vi "data insert core.vi"(8 "error in (no error)":errorcluster, 9 "column information":T1[](array[typedef]), 10 "data":variant[](array[variant]), 11 "table":string) -> (0 "error out":errorcluster)   [LabVIEW 2016, in "斯坦道多参数.lvlib"]
uses:
  <vilib>/addons/database/Auxilliary.llb/DB Tools Column Info.ctl
  <vilib>/addons/database/Auxilliary.llb/DB Tools DataTypes.ctl
  <vilib>/Utility/sysdir.llb/System Directory Type.ctl
  <vilib>/addons/database/Auxilliary.llb/DB Tools Transaction.ctl
  <vilib>/addons/database/Auxilliary.llb/DB Tools Isolation Level.ctl
  <vilib>/addons/database/Auxilliary.llb/DB Tools Parameter Info.ctl
  <vilib>/addons/database/Auxilliary.llb/DB Tools Parameter Dir.ctl
  <vilib>/addons/database/Connection.llb/DB Tools Open Connec (String).vi
  <vilib>/addons/database/Connection.llb/Conn Transaction.vi
  <vilib>/addons/database/Connection.llb/Conn Execute.vi
  <vilib>/addons/database/Recordset.llb/Rec Destroy - Connection.vi
  <vilib>/addons/database/Command.llb/Cmd Set Parameter Value (C).vi
  <vilib>/addons/database/Auxilliary.llb/DB Tools Format Datetime String (Time Stamp).vi
  <vilib>/addons/database/Command.llb/Cmd Execute.vi
  <vilib>/addons/database/Recordset.llb/Rec Destroy - Command.vi
  <vilib>/addons/database/Command.llb/Cmd Delete.vi
  <vilib>/addons/database/NI_Database_API.lvlib
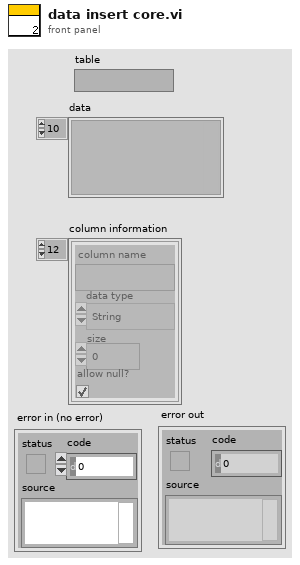
[diagram p1: front panel]
types:
  T1 = typedef "NI_Database_API.lvlib/DB Tools Column Info.ctl" = cluster{"column name":string, "data type":T2, "size":i32, "allow null?":bool}
  T2 = typedef "NI_Database_API.lvlib/DB Tools DataTypes.ctl" = enum16{"String", "Long (I32)", "Single (SGL)", "Double (DBL)", "Date/Time", "Binary"}
  T3 = typedef "NI_Database_API.lvlib/DB Tools Isolation Level.ctl" = enum16{"chaos", "read uncommitted", "read committed", "repeatable read", "serializable"}
  T4 = typedef "NI_Database_API.lvlib/DB Tools Transaction.ctl" = enum16{"begin", "commit", "rollback"}
  T5 = typedef "System Directory Type.ctl" = i32
  T6 = typedef "NI_Database_API.lvlib/Conn ObjectReference.ctl" = refnum<k1>
  T7 = typedef "NI_Database_API.lvlib/DB Tools Parameter Info.ctl" = cluster{"parameter name":string, "type":T2, "direction":T8, "value":variant}
  T8 = typedef "NI_Database_API.lvlib/DB Tools Parameter Dir.ctl" = enum32{"Input", "Output", "Input/Output", "Return Value"}
  T9 = typedef "NI_Database_API.lvlib/Rec ObjectReference.ctl" = refnum<k1>
  T10 = typedef "NI_Database_API.lvlib/Cmd ObjectReference.ctl" = refnum<k1>
  T11 = typedef "NI_Database_API.lvlib/Cmd-Rec Object Reference.ctl" = refnum<k1>
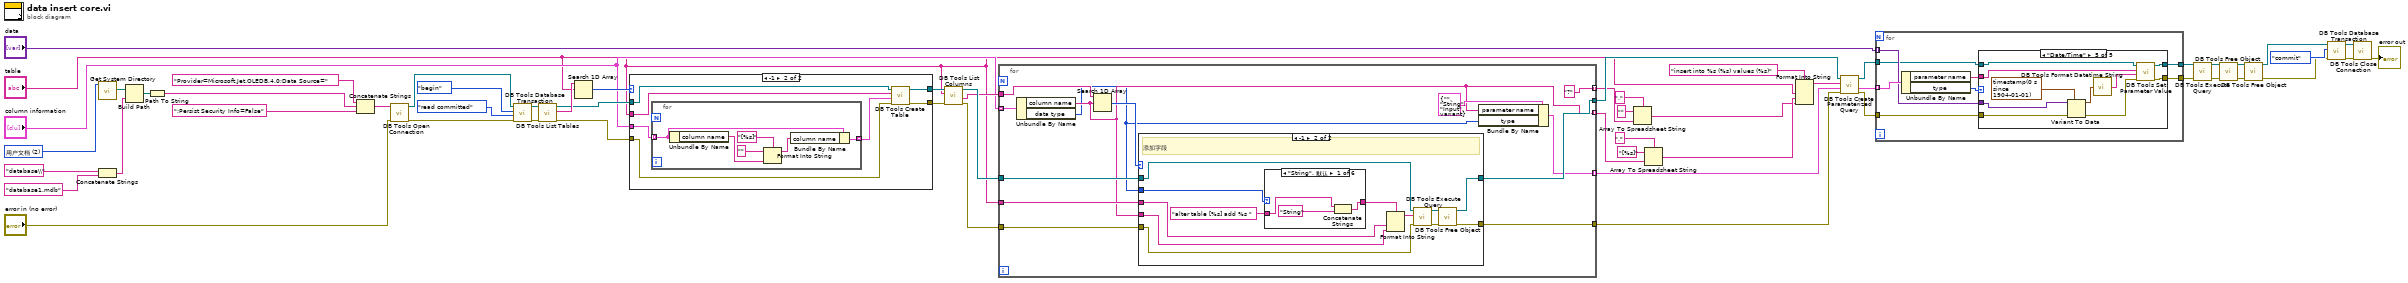
[diagram p0: block diagram]
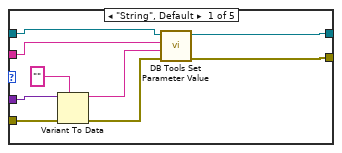
[diagram p2: hidden frame]
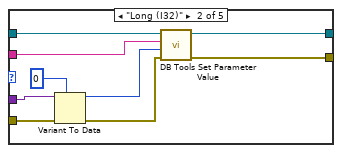
[diagram p3: hidden frame]
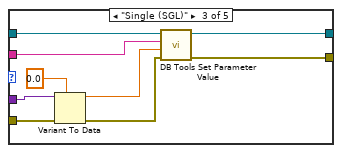
[diagram p4: hidden frame]
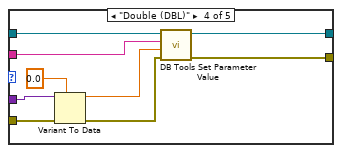
[diagram p5: hidden frame]
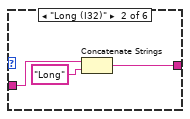
[diagram p7: hidden frame]
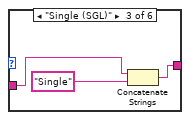
[diagram p8: hidden frame]
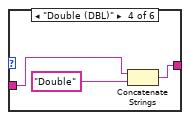
[diagram p9: hidden frame]
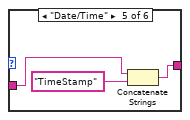
[diagram p10: hidden frame]
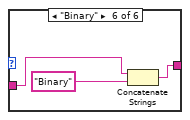
[diagram p11: hidden frame]
diagram:
  w57 = T5 2 items=["用户目录"=0, "用户桌面"=1, "用户文档"=2, "用户应用程序数据"=3, "用户设置"=4, "用户临时目录"=5, "公共文档"=6, "公共应用程序数据"=7, "公共设置"=8, "公共缓存"=13, "系统核心库"=9, "系统安装库"=10, "应用程序文件"=11, "启动盘根目录"=12] ("system directory type")
  n1 = call <vilib>:"Get System Directory.vi"("system directory type"=w57) -> ("system directory"=w55:path)  [unwired: 10 in]
  n2 = Concatenate Strings("database\\" ("condition"), "database1.mdb" ("database")) -> (w49:string)
  n3 = Build Path(base path=w55, name or relative path=w49) -> (appended path=w54:path)
  n4 = Path To String(path=w54) -> (string=w53:string)
  n5 = Concatenate Strings("Provider=Microsoft.Jet.OLEDB.4.0;Data Source=" ("condition"), w53, ";Persist Security Info=False" ("condition")) -> (w51:string)
  n6 = call-poly <vilib>:"DB Tools Open Connection.vi"("error in (no error)"="error in (no error)", "connection information"=w51) -> ("error out"=w3:errorcluster, "connection reference"=w5:T6)  [unwired: 6 in]
  n7 = call-poly <vilib>:"DB Tools Database Transaction.vi"("error in (no error)"=w3, "isolation level (chaos)"=DB_Tools_Isolation_Level."read committed", "operation (begin)"=DB_Tools_Transaction."begin", "connection reference"=w5) -> ("error out"=w2:errorcluster, "connection reference out"=w4:T6)  [unwired: 2 in]
  n8 = call <vilib>:"DB Tools List Tables.vi"("error in (no error)"=w2, "connection reference"=w4) -> ("error out"=w39:errorcluster, "tables"=w42:string[], "connection reference out"=w40:T6)  [unwired: 3 in]
  n9 = Search 1D Array(1D array=w42, element="table") -> (index of element=w41:i32)  [unwired: 1 in]
  n10 = case shown="-1" w41 {
    tunnel: w40 -> [w59 w66]
    tunnel: w39 -> [w58 w65]
    tunnel: "table" -> [_ w64]
    tunnel: "column information" -> [_ w61]
    tunnel: [w59 w63] -> w34
    tunnel: [w58 w62] -> w33
    frame 0, Default {
    }
    frame -1 {
      n11 = for {
        tunnel: w61 -> [w68] mode=indexing
        tunnel: [w67] -> w60 mode=indexing
        n12 = Unbundle By Name(w68) -> ("column name"=w72:string)
        n13 = Format Into String(format string="[%s]" ("格式字符串"), initial string="" ("初始字符串"), w72) -> (resulting string=w69:string)  [unwired: 1 in, 1 out]
        n14 = Bundle By Name(cluster=w68, "column name"=w69) -> (w67:T1)
      }
      n15 = call <vilib>:"DB Tools Create Table.vi"("error in (no error)"=w65, "column information"=w60, "table"=w64, "connection reference"=w66) -> ("error out"=w62:errorcluster, "connection reference out"=w63:T6)  [unwired: 4 in]
    }
  }
  n16 = call <vilib>:"DB Tools List Columns.vi"("error in (no error)"=w33, "table"="table", "connection reference"=w34) -> ("error out"=w36:errorcluster, "columns"=w37:string[], "connection reference out"=w38:T6)  [unwired: 1 in, 1 out]
  n17 = for {
    tunnel: w38 -> [w83]
    tunnel: w37 -> [w85]
    tunnel: w36 -> [w82]
    tunnel: [w81] -> w32
    tunnel: [w80] -> w31
    tunnel: "table" -> [w79]
    tunnel: "column information" -> [w78] mode=indexing
    tunnel: [w76] -> w30 mode=indexing
    tunnel: [w75] -> w23 mode=indexing
    tunnel: ["?"] -> w21 mode=indexing
    n18 = Unbundle By Name(w78) -> ("column name"=w75:string, "data type"=w73:T2)
    n19 = Search 1D Array(1D array=w85, element=w75) -> (index of element=w84:i32)  [unwired: 1 in]
    n20 = case shown="-1" w84 {
      tunnel: [w87 w96] -> w80
      tunnel: [w86 w95] -> w81
      tunnel: w83 -> [w87 w94]
      tunnel: w75 -> [_ w93]
      tunnel: w82 -> [w86 w92]
      tunnel: w79 -> [_ w91]
      tunnel: w73 -> [_ w89]
      frame 0, Default {
      }
      frame -1 {
        # "添加字段"
        n21 = case shown="\"String\", 默认" w89 {
          tunnel: "alter table [%s] add %s " -> [w102 w105 w108 w111 w114 w117]
          tunnel: [w101 w104 w107 w110 w113 w116] -> w88
          frame "String", Default {
            n22 = Concatenate Strings(w102, "String" ("字符串")) -> (w101:string)
          }
          frame "Long (I32)" {
            n23 = Concatenate Strings(w105, "Long" ("字符串")) -> (w104:string)
          }
          frame "Single (SGL)" {
            n24 = Concatenate Strings(w108, "Single" ("字符串")) -> (w107:string)
          }
          frame "Double (DBL)" {
            n25 = Concatenate Strings(w111, "Double" ("字符串")) -> (w110:string)
          }
          frame "Date/Time" {
            n26 = Concatenate Strings(w114, "TimeStamp" ("字符串")) -> (w113:string)
          }
          frame "Binary" {
            n27 = Concatenate Strings(w117, "Binary" ("字符串")) -> (w116:string)
          }
        }
        n28 = Format Into String(format string=w88, w91, w93) -> (resulting string=w97:string)  [unwired: 2 in, 1 out]
        n29 = call-poly <vilib>:"DB Tools Execute Query.vi"("error in (no error)"=w92, "SQL query"=w97, "connection reference"=w94) -> ("error out"=w98:errorcluster, "recordset reference"=w99:T9)  [unwired: 5 in]
        n30 = call-poly <vilib>:"DB Tools Free Object.vi"("error in (no error)"=w98, "recordset reference"=w99) -> ("error out"=w95:errorcluster, "connection reference"=w96:T6)  [unwired: 8 in]
      }
    }
    n31 = Bundle By Name(cluster=T7 {"parameter name"="", "type"=enum."String", "direction"=enum."Input", "value"=variant} ("parameter information"), "parameter name"=w75, "type"=w73) -> (w76:T7)
  }
  n32 = Array To Spreadsheet String(delimiter (Tab)="," ("分隔符(Tab)"), array=w21, 3:"" ("格式字符串")) -> (spreadsheet string=w20:string)
  n33 = Array To Spreadsheet String(delimiter (Tab)="," ("分隔符(Tab)"), array=w23, 3:"[%s]" ("格式字符串")) -> (spreadsheet string=w22:string)
  n34 = Format Into String(format string="insert into %s (%s) values (%s)" ("格式字符串"), "table", w22, w20) -> (resulting string=w19:string)  [unwired: 2 in, 1 out]
  n35 = call <vilib>:"DB Tools Create Parameterized Query.vi"("error in (no error)"=w32, "parameters"=w30, "SQL query"=w19, "connection reference"=w31) -> ("error out"=w17:errorcluster, "parameters out"=w16:T7[], "command reference"=w18:T10)  [unwired: 3 in]
  n36 = for {
    tunnel: w18 -> [w122]
    tunnel: w17 -> [w120]
    tunnel: w16 -> [w125] mode=indexing
    tunnel: "data" -> [w123] mode=indexing
    tunnel: [w119] -> w15
    tunnel: [w118] -> w14
    n37 = Unbundle By Name(w125) -> ("parameter name"=w121:string, "type"=w124:T2)
    n38 = case shown="\"Date/Time\"" w124 {
      tunnel: w123 -> [w129 w137 w144 w154 w171]
      tunnel: w122 -> [w132 w141 w148 w158 w169]
      tunnel: w121 -> [w131 w140 w147 w153 w168]
      tunnel: w120 -> [w126 w135 w145 w155 w166]
      tunnel: [w128 w139 w149 w157 w165] -> w119
      tunnel: [w127 w138 w146 w156 w164] -> w118
      frame "String", Default {
        n39 = Variant To Data(error in=w126, type="", Variant=w129) -> (data=w130:string, error out=w134:errorcluster)
        n40 = call-poly <vilib>:"DB Tools Set Parameter Value.vi"("error in (no error)"=w134, "value"=w130, "parameter index"=w131, "command reference"=w132) -> ("error out"=w127:errorcluster, "command reference out"=w128:T10)  [unwired: 4 in]
      }
      frame "Long (I32)" {
        n41 = Variant To Data(error in=w135, type=0, Variant=w137) -> (data=w142:i32, error out=w143:errorcluster)
        n42 = call-poly <vilib>:"DB Tools Set Parameter Value.vi"("error in (no error)"=w143, "value"=w142, "parameter index"=w140, "command reference"=w141) -> ("error out"=w138:errorcluster, "command reference out"=w139:T10)  [unwired: 4 in]
      }
      frame "Single (SGL)" {
        n43 = Variant To Data(error in=w145, type=sgl 0.0, Variant=w144) -> (data=w151:sgl, error out=w152:errorcluster)
        n44 = call-poly <vilib>:"DB Tools Set Parameter Value.vi"("error in (no error)"=w152, "value"=w151, "parameter index"=w147, "command reference"=w148) -> ("error out"=w146:errorcluster, "command reference out"=w149:T10)  [unwired: 4 in]
      }
      frame "Double (DBL)" {
        n45 = Variant To Data(error in=w155, type=0.0, Variant=w154) -> (data=w160:dbl, error out=w161:errorcluster)
        n46 = call-poly <vilib>:"DB Tools Set Parameter Value.vi"("error in (no error)"=w161, "value"=w160, "parameter index"=w153, "command reference"=w158) -> ("error out"=w156:errorcluster, "command reference out"=w157:T10)  [unwired: 4 in]
      }
      frame "Date/Time" {
        n47 = Variant To Data(error in=w166, type=timestamp(0 s since 1904-01-01) ("时间标识"), Variant=w171) -> (data=w163:timestamp, error out=w167:errorcluster)
        n48 = call-poly <vilib>:"DB Tools Format Datetime String.vi"("time stamp"=w163) -> ("date/time string"=w162:string)
        n49 = call-poly <vilib>:"DB Tools Set Parameter Value.vi"("error in (no error)"=w167, "value"=w162, "parameter index"=w168, "command reference"=w169) -> ("error out"=w164:errorcluster, "command reference out"=w165:T10)  [unwired: 4 in]
      }
    }
  }
  n50 = call-poly <vilib>:"DB Tools Execute Query.vi"("error in (no error)"=w14, "command reference"=w15) -> ("error out"=w12:errorcluster, "command-recordset reference"=w13:T11)  [unwired: 6 in]
  n51 = call-poly <vilib>:"DB Tools Free Object.vi"("error in (no error)"=w12, "command-recordset reference"=w13) -> ("error out"=w10:errorcluster, "command reference"=w11:T10)  [unwired: 8 in]
  n52 = call-poly <vilib>:"DB Tools Free Object.vi"("error in (no error)"=w10, "command reference"=w11) -> ("error out"=w6:errorcluster, "connection reference"=w7:T6)  [unwired: 8 in]
  n53 = call-poly <vilib>:"DB Tools Database Transaction.vi"("error in (no error)"=w6, "operation (begin)"=DB_Tools_Transaction."commit", "connection reference"=w7) -> ("error out"=w8:errorcluster, "connection reference out"=w9:T6)  [unwired: 3 in]
  n54 = call <vilib>:"DB Tools Close Connection.vi"("error in (no error)"=w8, "connection reference"=w9) -> ("error out"=→"error out":errorcluster)  [unwired: 5 in]
